vi "vi open_close.vi"(8 "error in":errorcluster, 10 "Path":path, 11 "Enum":enum16{"Open", "Close"}(ring)=enum."Close") -> (0 "error out":errorcluster)   [LabVIEW 2012]
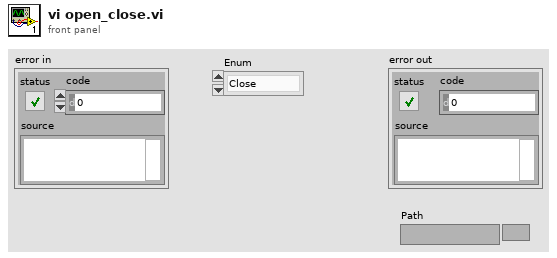
[diagram p1: front panel]
types:
  T1 = enum32{"Invalid", "Standard", "Closed", "Hidden", "Minimized", "Maximized"}
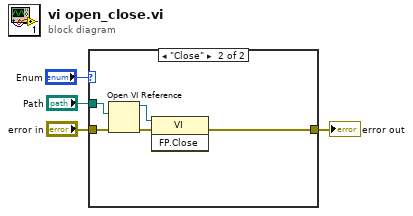
[diagram p0: block diagram]
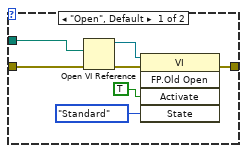
[diagram p2: hidden frame]
diagram:
  n1 = case shown="\"Close\"" "Enum" {
    tunnel: "Path" -> [w7 w15]
    tunnel: "error in" -> [w5 w14]
    tunnel: [w6 w13] -> w1
    frame "Open", Default {
      n2 = Open VI Reference(vi path=w7, error in (no error)=w5) -> (vi reference=w10:refnum<vi>, error out=w11:errorcluster)  [unwired: 1 in, 3 out]
      n3 = invoke class="VI" method="FP.Old Open"(reference=w10, error in=w11, "Activate"=TRUE, "State"=T1."Standard") -> (error out=w6:errorcluster)  [unwired: 1 in, 4 out]
    }
    frame "Close" {
      n4 = Open VI Reference(vi path=w15, error in (no error)=w14) -> (vi reference=w12:refnum<vi>, error out=w16:errorcluster)  [unwired: 1 in, 3 out]
      n5 = invoke class="VI" method="FP.Close"(reference=w12, error in=w16) -> (error out=w13:errorcluster)  [unwired: 1 in, 2 out]
    }
  }
  "error out" <- w1
